vi "Extract Port From Host String.vi"(0 "host in":string) -> (4 "host out":string, 6 "port":u16, 8 "found?":bool)   [LabVIEW 2013, in "AMC.lvlib"]
uses:
  AMC.lvlib
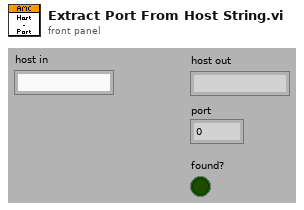
[diagram p1: front panel]
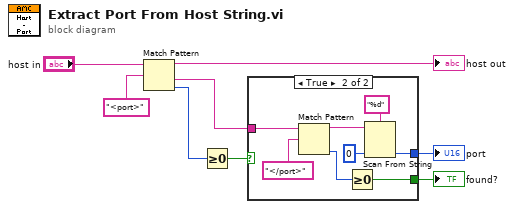
[diagram p0: block diagram]
diagram:
  n1 = Match Pattern(string="host in", regular expression="<port>" ("string")) -> (before substring=→"host out":string, after substring=w8:string, offset past match=w7:i32)  [unwired: 1 in, 1 out]
  n2 = Greater Or Equal To 0?(x=w7) -> (x >= 0?=w6:bool)
  n3 = case shown="True" w6 {
    tunnel: w8 -> [_ w12]
    tunnel: [_ w11] -> w2
    tunnel: [_ w9] -> w1
    frame False {
    }
    frame True {
      n4 = Match Pattern(string=w12, regular expression="</port>" ("string")) -> (before substring=w14:string, offset past match=w10:i32)  [unwired: 1 in, 2 out]
      n5 = Greater Or Equal To 0?(x=w10) -> (x >= 0?=w9:bool)
      n6 = Scan From String(format string="%d", input string=w14, default 1=u16 0 ("default value 1")) -> (output 1=w11:u16)  [unwired: 2 in, 3 out]
    }
  }
  "port" <- w2
  "found?" <- w1
